vi "C(T) data packer.vi"(0 "Path in":path=path "C:/Documents and Settings/pk/My Documents/P350/P350 F01/P350 F01 Instructor/Projects w sol/P5/P350 C(T) experimental data file 11 06 01 c.txt", 1 "launch viewer":bool=TRUE, 5 "Temp Array In":dbl[](array[numeric])=[26.0, 30.0, 34.0, 38.0, 42.0, 46.0, 50.0] format="%.2f", 7 "Timing Control Parameters In":T1={"N cycles for averaging"=100, "N points per measurement"=1000, "Measurment time interval"=2e-05} {"Measurment time interval" format="%.2e"}, 9 "Data In":waveform(dbl)[](array[waveform])=[{"t0"=timestamp(3087922235.213 s since 1904-01-01), "dt"=1.9999999494757503e-05, "Y"=array[1000 elements]}, {"t0"=timestamp(3087922405.147 s since 1904-01-01), "dt"=1.9999999494757503e-05, "Y"=array[1000 elements]}, {"t0"=timestamp(3087922549.515 s since 1904-01-01), "dt"=1.9999999494757503e-05, "Y"=array[1000 elements]}, {"t0"=timestamp(3087922690.9379997 s since 1904-01-01), "dt"=1.9999999494757503e-05, "Y"=array[1000 elements]}, {"t0"=timestamp(3087922829.417 s since 1904-01-01), "dt"=1.9999999494757503e-05, "Y"=array[1000 elements]}, {"t0"=timestamp(3087922967.796 s since 1904-01-01), "dt"=1.9999999494757503e-05, "Y"=array[1000 elements]}, {"t0"=timestamp(3087923101.799 s since 1904-01-01), "dt"=1.9999999494757503e-05, "Y"=array[1000 elements]}], 11 "error in":errorcluster) -> (4 "Path out":path=path "C:/Documents and Settings/pk/My Documents/P350/P350 F01/P350 F01 Instructor/Projects w sol/P5/P350 C(T) experimental data file 11 06 01 c.txt", 8 "data spreadsheet":dbl[][](array[numeric]) format="%.2e", 13 "no save out":bool, 15 "error out":errorcluster)   [LabVIEW 2016]
doc: "This vi manages the data processing and data viewing process after acquisition.\n\nPaul K Dixon\nPhysics 350\nCSUSB Physics"
uses:
  globals/C(T) global variables.vi
panel:
  in  "Resistance (Ohms)":dbl=100000.0 format="%.4e"
  out "N temps":i32=7
  # "C(T) Data Packer"
  # "t params"
  # "N temps"
  # "temps"
  # "est caps"
  # "RC decays - - - - - -"
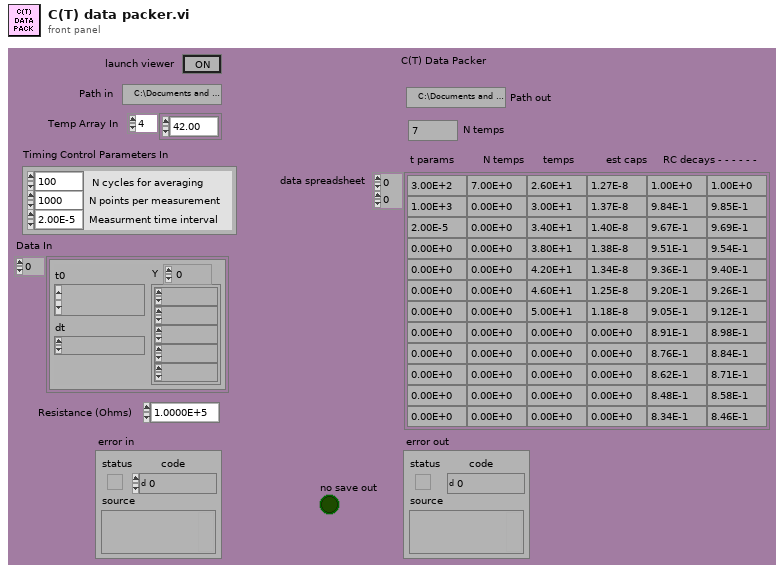
[diagram p1: front panel]
types:
  T1 = cluster{"N cycles for averaging":i32, "N points per measurement":i32, "Measurment time interval":dbl}
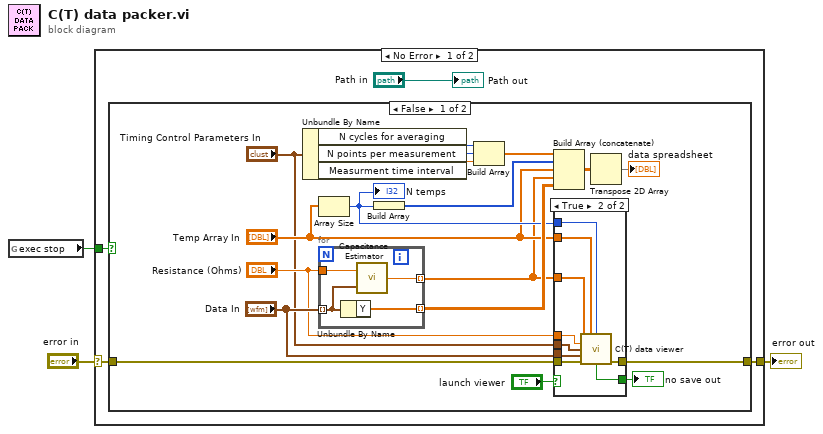
[diagram p0: block diagram]
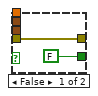
[diagram p2: hidden frame]
diagram:
  n1 = global read "C(T) global variables.vi" "exec stop"() -> (w1:bool)
  n2 = case shown="No Error" "error in" {
    selector: "error in" -> [w7 w42]
    tunnel: [w6 w42] -> w2
    tunnel: w1 -> [w4 _]
    frame No Error {
      n3 = case shown="False" w4 {
        tunnel: w7 -> [w11 w41]
        tunnel: [w10 w41] -> w6
        frame False {
          n4 = Unbundle By Name("Timing Control Parameters In") -> ("N cycles for averaging"=w23:i32, "N points per measurement"=w24:i32, "Measurment time interval"=w25:dbl)
          n5 = Array Size(array="Temp Array In") -> (size(s)=w16:i32)
          "N temps" <- w16
          n6 = for {
            tunnel: "Data In" -> [w39] mode=indexing
            tunnel: [w40] -> w18 mode=indexing
            tunnel: "Resistance (Ohms)" -> [w38]
            tunnel: [w37] -> w14 mode=indexing
            n7 = Unbundle By Name(w39) -> ("Y"=w40:dbl[])
            n8 = call "Capacitance Estimator.vi"("normalized waveform"=w39, "Resistance (Ohms)"=w38) -> ("Estimated Capacitance (F)"=w37:dbl)
          }
          n9 = Build Array(w16) -> (w19:i32[])
          n10 = Build Array(w23, w24, w25) -> (w20:dbl[])
          n11 = Build Array (concatenate)(w20, w19, "Temp Array In", w14, w18) -> (w22:dbl[][])
          n12 = case shown="True" "launch viewer" {
            tunnel: "Data In" -> [_ w36]
            tunnel: w16 -> [_ w35]
            tunnel: "Temp Array In" -> [_ w34]
            tunnel: w14 -> [_ w33]
            tunnel: "Resistance (Ohms)" -> [_ w32]
            tunnel: "Timing Control Parameters In" -> [_ w31]
            tunnel: w11 -> [w27 w30]
            tunnel: [w27 w29] -> w10
            tunnel: [FALSE ("no save out") w28] -> w8
            frame False {
            }
            frame True {
              n13 = call "C(T) data viewer.vi"("Cap Estimates"=w33, "Temps"=w34, "N Temps"=w35, "Resistance (Ohms)"=w32, "Timing Control Parameters"=w31, "waveforms"=w36, "error in"=w30) -> ("no save out"=w28:bool, "error out"=w29:errorcluster)  [unwired: 7 out]
            }
          }
          "no save out" <- w8
          n14 = Transpose 2D Array(2D array=w22) -> (transposed array=→"data spreadsheet":dbl[][])
        }
        frame True {
        }
      }
      "Path out" <- "Path in"
    }
    frame Error {
    }
  }
  "error out" <- w2
